vi "rad_Configure Application Image.vi"(7 "Temp Folder":path, 8 "error in (no error)":errorcluster, 11 "App Images Information":T1) -> (0 "error out":errorcluster, 2 "Cancelled":bool, 3 "App Images Information":T1)   [LabVIEW 2020]
uses:
  TypeDefs/rad_AppImage Information.ctl
  TypeDefs/rad_Application Image Properties.ctl
  TypeDefs/rad_FPGA Properties.ctl
  TypeDefs/rad_FPGA Flash Properties.ctl
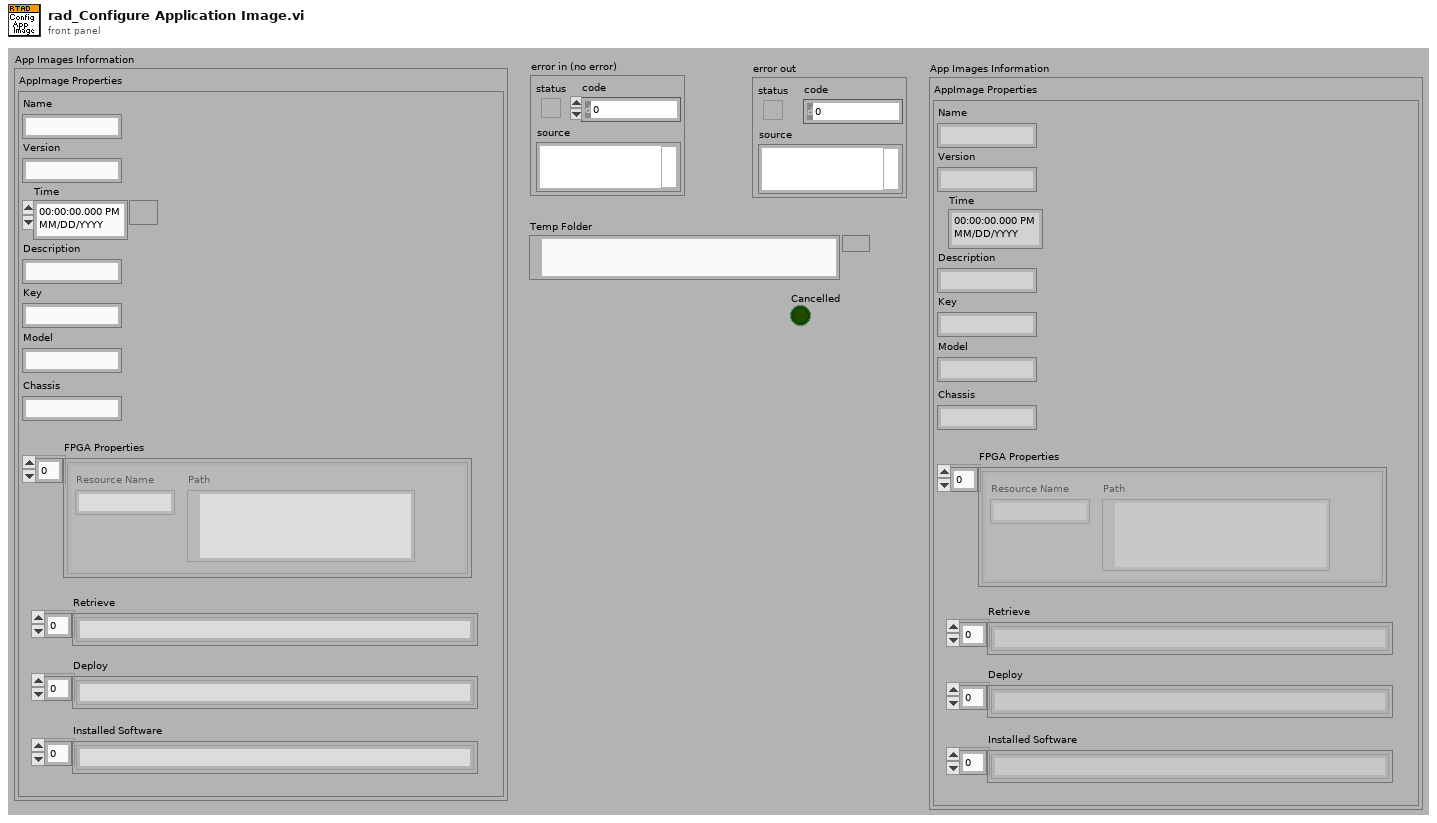
[diagram p1: front panel]
types:
  T1 = typedef "rad_AppImage Information.ctl" = cluster{"AppImage Properties":T2, "AppImage Path":path}
  T2 = typedef "rad_Application Image Properties.ctl" = cluster{"Name":string, "Version":string, "Time":timestamp, "Description":string, "Key":string, "Chassis":string, "FPGA Properties":T3, "Model":string, "Retrieve":string[], "Deploy":string[], "Installed Software":string[]}
  T3 = typedef "rad_FPGA Properties.ctl" = T4[]
  T4 = typedef "rad_FPGA Flash Properties.ctl" = cluster{"Resource Name":string, "Path":path}
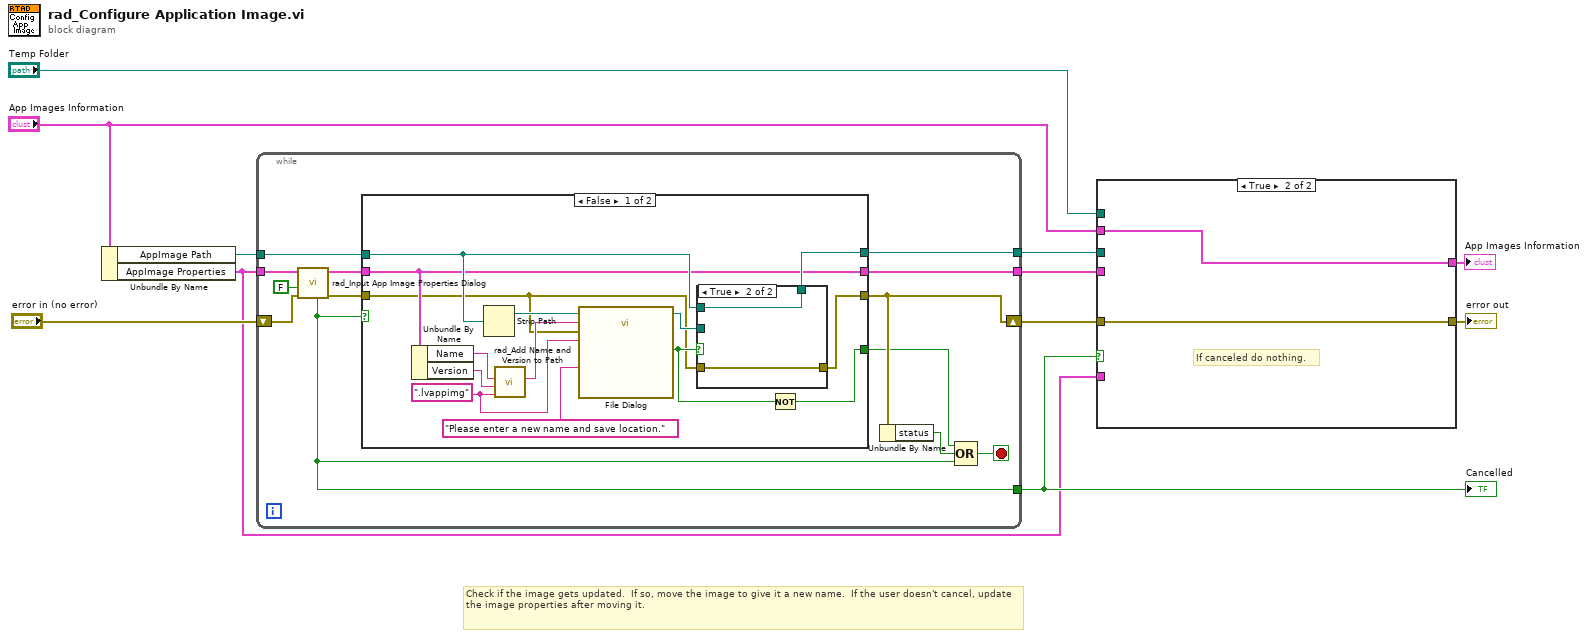
[diagram p0: block diagram]
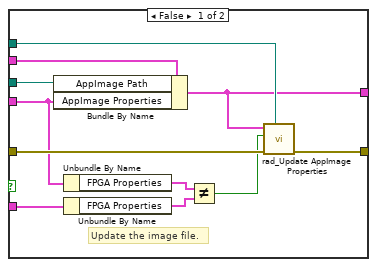
[diagram p2: hidden frame]
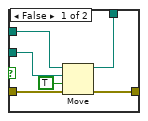
[diagram p3: hidden frame]
diagram:
  # "Check if the image gets updated.  If so, move the image to give it a new name.  If the user doesn't cancel, update the image properties after moving it."
  n1 = Unbundle By Name("App Images Information") -> ("AppImage Path"=w6:path, "AppImage Properties"=w3:T2)
  n2 = while {
    shift-right: [w16] -> w9
    shift-left: "error in (no error)" -> [w22]
    tunnel: [w14] -> w10
    tunnel: [w13] -> w7
    tunnel: w6 -> [w12]
    tunnel: w3 -> [w23]
    tunnel: [w19] -> w8
    stop <- w17 stop-if-true
    n3 = call "rad_Input App Image Properties Dialog.vi"("error in (no error)"=w22, "New Image?"=FALSE, "AppImage Properties"=w23) -> ("error out"=w21:errorcluster, "AppImage Properties"=w20:T2, "Cancelled"=w14:bool)  [unwired: 6 in]
    n4 = case shown="False" w14 {
      tunnel: w21 -> [w25 w48]
      tunnel: w20 -> [w31 w47]
      tunnel: [w31 w47] -> w19
      tunnel: [w38 w48] -> w16
      tunnel: [w33 _] -> w15
      tunnel: [w37 _] -> w13
      tunnel: w12 -> [w35 _]
      frame False {
        w27 = ".lvappimg" ("File Extension")
        n5 = Unbundle By Name(w31) -> ("Name"=w30:string, "Version"=w29:string)
        n6 = Strip Path(path=w35) -> (stripped path=w36:path)  [unwired: 1 out]
        n7 = call "rad_Add Name and Version to Path.vi"("File Extension"=w27, "Version"=w29, "Name"=w30) -> ("filename without extension"=w28:string)  [unwired: 7 in, 1 out]
        n8 = call "File Dialog"("start path"=w36, "prompt"="Please enter a new name and save location.", "default name"=w28, "error in"=w25, "pattern (all files)"=w27) -> ("selected path"=w32:path, "cancelled"=w34:bool)  [unwired: 7 in, 2 out]
        n9 = case shown="True" w34 {
          tunnel: [w44 w45] -> w38
          tunnel: [w42 w46] -> w37
          tunnel: w25 -> [w41 w45]
          tunnel: w35 -> [w40 w46]
          tunnel: w32 -> [w39 _]
          frame False {
            n10 = Move(source path=w40, error in=w41, 9:TRUE ("overwrite (F)"), 10:w39) -> (error out=w44:errorcluster, 3:w42:path)  [unwired: 1 in, 1 out]
          }
          frame True {
          }
        }
        n11 = Not(x=w34) -> (.not. x?=w33:bool)
      }
      frame True {
      }
    }
    n12 = Unbundle By Name(w16) -> ("status"=w18:bool)
    n13 = Compound Arithmetic op=OR(w15, w18, w14) -> (w17:bool)
  }
  "Cancelled" <- w10
  n14 = case shown="True" w10 {
    tunnel: w9 -> [w59 w61]
    tunnel: w8 -> [w53 _]
    tunnel: w7 -> [w57 _]
    tunnel: "App Images Information" -> [w58 w60]
    tunnel: "Temp Folder" -> [w56 _]
    tunnel: w3 -> [w52 _]
    tunnel: [w50 w61] -> w2
    tunnel: [w49 w60] -> w1
    frame False {
      # "Update the image file."
      n15 = Bundle By Name(cluster=w58, "AppImage Path"=w57, "AppImage Properties"=w53) -> (w49:T1)
      n16 = Unbundle By Name(w53) -> ("FPGA Properties"=w54:T3)
      n17 = Unbundle By Name(w52) -> ("FPGA Properties"=w55:T3)
      n18 = Not Equal?(x=w54, y=w55) -> (x != y?=w51:bool)
      n19 = call "rad_Update AppImage Properties.vi"("Temp Folder"=w56, "error in (no error)"=w59, "Bitfiles Modified?"=w51, "AppImage Information"=w49) -> ("error out"=w50:errorcluster)  [unwired: 7 in]
    }
    frame True {
      # "If canceled do nothing."
    }
  }
  "error out" <- w2
  "App Images Information" <- w1
